vi "Read Data.vi"(8 "error in (no error)":errorcluster, 11 "Serial Config":T1={"串口选择"="", "通讯速率"=9600, "超时时间"=10000, "数据位长"=8, "奇偶校验"=enum."None", "停止位长"=10, "握手控制"=0, "字符结束"=TRUE, "结束字符"=10, "仪器地址"=1} {"结束字符" format="%.0x"; "握手控制" items=["None", "XON/XOFF", "RTS/CTS", "XON/XOFF & RTS/CTS", "DTR/DSR", "XON/XOFF & DTR/DSR"]; "停止位长" items=["1.0"=10, "1.5"=15, "2.0"=20]; "数据位长" min=5 max=8 step=1}) -> (0 "error out":errorcluster, 2 "Status":string, 3 "RV":dbl[](array[numeric]))   [LabVIEW 2010, in "CM51.lvlib"]
doc: "Use this template to build a VI to use as a subVI."
uses:
  CM51.lvlib
  Serial Config.ctl
  CM51Channel.ctl
  <vilib>/Instr/_visa.llb/VISA Configure Serial Port (Instr).vi
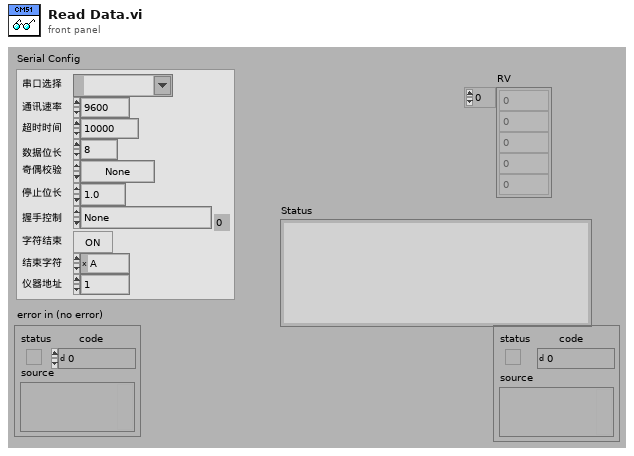
[diagram p1: front panel]
types:
  T1 = typedef "CM51.lvlib/Serial Config.ctl" = cluster{"串口选择":refnum<visa-resource-name>, "通讯速率":u32, "超时时间":u32, "数据位长":u16, "奇偶校验":enum16{"None", "Odd", "Even", "Mark", "Space"}, "停止位长":u16, "握手控制":u16, "字符结束":bool, "结束字符":u8, "仪器地址":u32}
  T2 = typedef "CM51.lvlib/CM51Channel.ctl" = enum16{"RV1", "RV2", "RV3"}
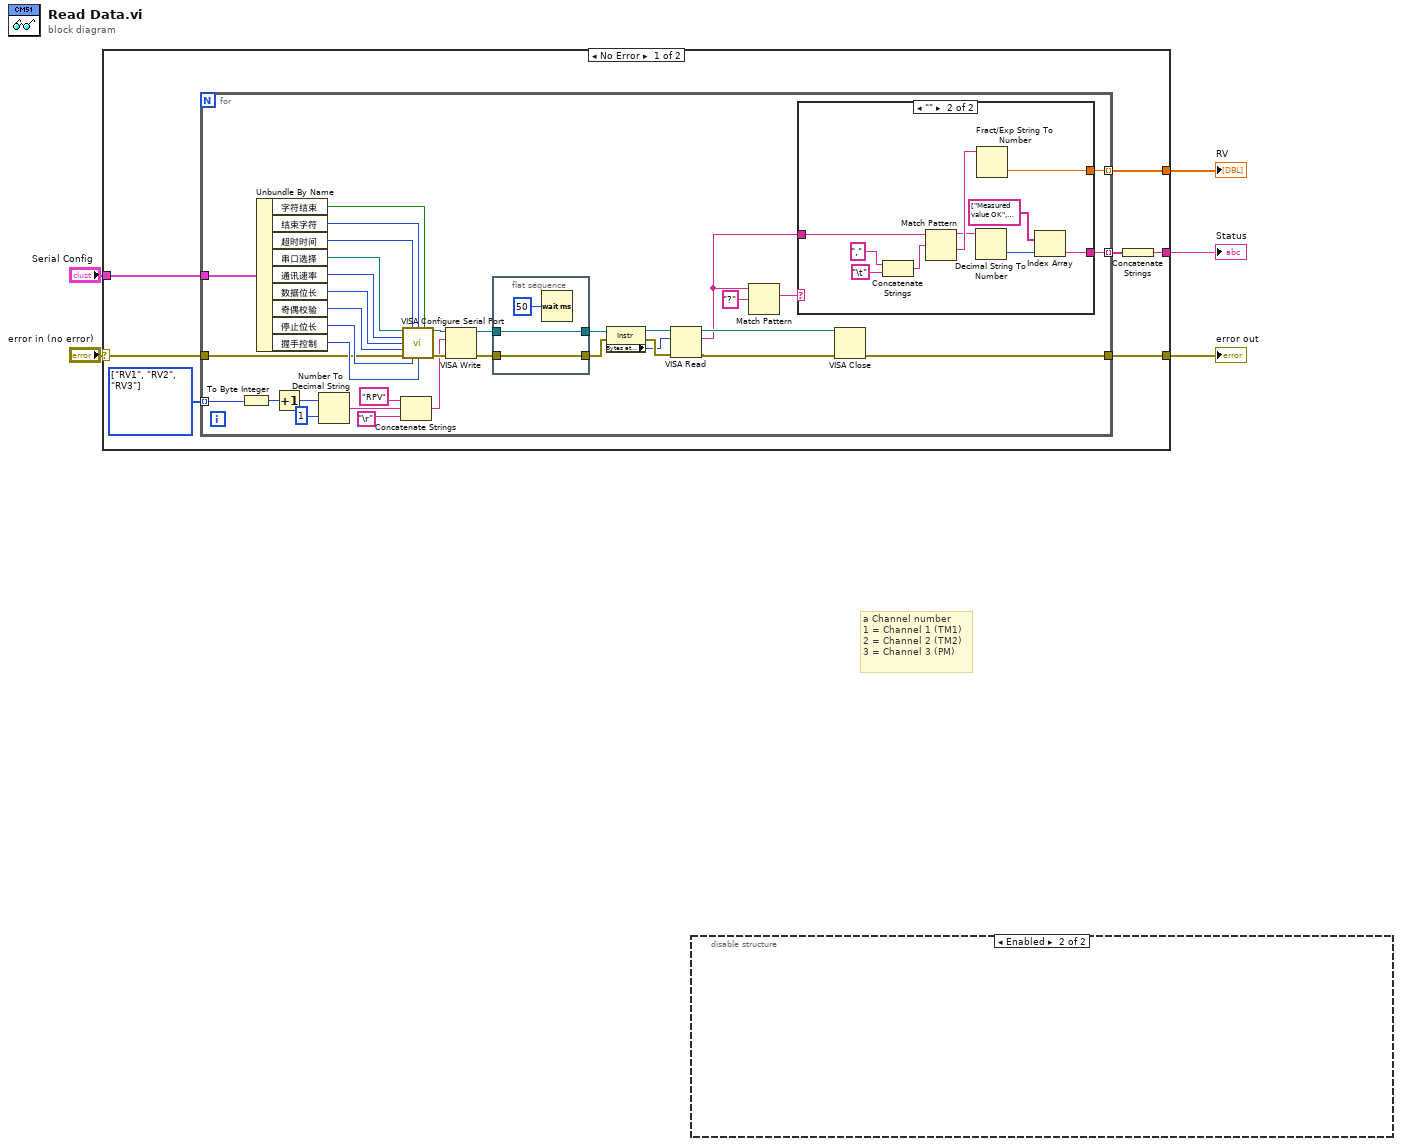
[diagram p0: block diagram]
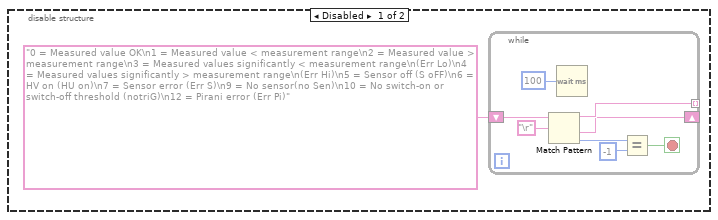
[diagram p2: hidden frame]
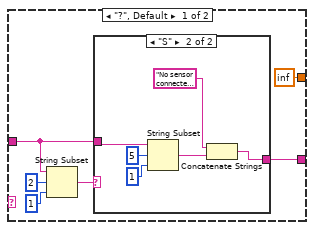
[diagram p3: hidden frame]
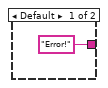
[diagram p4: hidden frame]
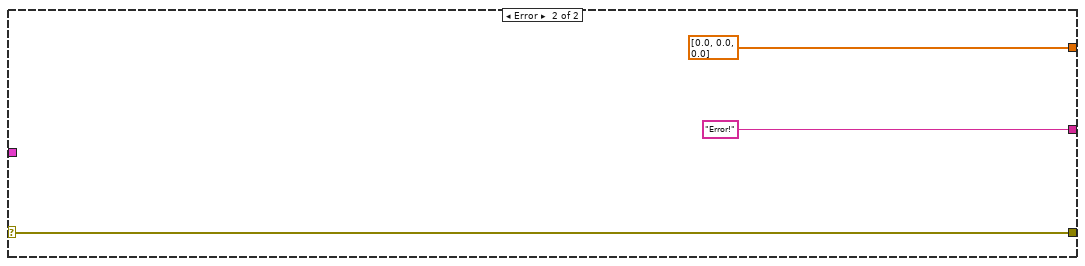
[diagram p5: hidden frame]
diagram:
  # "a Channel number\n1 = Channel 1 (TM1)\n2 = Channel 2 (TM2)\n3 = Channel 3 (PM)"
  n1 = case shown="No Error" "error in (no error)" {
    selector: "error in (no error)" -> [w11 w77]
    tunnel: [w10 w77] -> w4
    tunnel: "Serial Config" -> [w12 _]
    tunnel: [w6 "Error!"] -> w1
    tunnel: [w8 dbl[] [0.0, 0.0, 0.0]] -> w2
    frame No Error {
      w9 = T2[] [enum."RV1", enum."RV2", enum."RV3"] items=["RV1", "RV2", "RV3"]
      n2 = for {
        tunnel: w12 -> [w46]
        tunnel: w11 -> [w36]
        tunnel: [w35] -> w10
        tunnel: w9 -> [w28] mode=indexing
        tunnel: [w27] -> w7 mode=indexing
        tunnel: [w26] -> w8 mode=indexing
        n3 = To Byte Integer(number=w28) -> (8bit integer=w34:i8)
        n4 = Unbundle By Name(w46) -> ("字符结束"=w41:bool, "结束字符"=w42:u8, "超时时间"=w43:u32, "串口选择"=w45:refnum<visa-resource-name>, "通讯速率"=w44:u32, "数据位长"=w40:u16, "奇偶校验"=w39:enum16{"None", "Odd", "Even", "Mark", "Space"}, "停止位长"=w38:u16, "握手控制"=w37:u16)
        n5 = Increment(x=w34) -> (x+1=w33:i8)
        n6 = Number To Decimal String(number=w33, width (-)=i16 1 ("宽度(-)")) -> (decimal integer string=w30:string)
        n7 = Concatenate Strings("RPV" ("字符串"), w30, "\r") -> (w16:string)
        n8 = call-poly "VISA Configure Serial Port"("VISA resource name"=w45, "timeout (10sec)"=w43, "termination char\n(0xA = '\\n' = LF)"=w42, "Enable Termination\nChar (T)"=w41, "baud rate (9600)"=w44, "data bits (8)"=w40, "parity (0:none)"=w39, "error in (no error)"=w36, "stop bits (10: 1 bit)"=w38, "flow control (0:none)"=w37) -> ("VISA resource name out"=w47:refnum<visa-resource-name>, "error out"=w48:errorcluster)  [unwired: 4 in]
        n9 = VISA Write(VISA resource name=w47, write buffer=w16, error in (no error)=w48) -> (VISA resource name out=w20:refnum<visa-resource-name>, error out=w19:errorcluster)  [unwired: 1 out]
        n10 = flat-sequence {
          tunnel: w20 -> [w74]
          tunnel: w19 -> [w73]
          tunnel: [w74] -> w18
          tunnel: [w73] -> w17
          frame #0 {
            n11 = Wait (ms)(milliseconds to wait=u32 50) -> ()  [unwired: 1 out]
          }
        }
        n12 = property class="Instr"(reference=w18, error in=w17) -> (reference out=w25:refnum<visa-resource-name>, error out=w23:errorcluster, "Bytes at Port"=w22:u32)
        n13 = VISA Read(VISA resource name=w25, byte count=w22, error in (no error)=w23) -> (VISA resource name out=w24:refnum<visa-resource-name>, read buffer=w15:string, error out=w21:errorcluster)  [unwired: 1 out]
        n14 = Match Pattern(string=w15, regular expression="?") -> (match substring=w13:string)  [unwired: 1 in, 3 out]
        n15 = case shown="\"\"" w13 {
          tunnel: [w50 w70] -> w27
          tunnel: [inf w69] -> w26
          tunnel: w15 -> [w49 w62]
          frame "?", Default {
            n16 = String Subset(string=w49, offset (0)=2, length (rest)=1 ("length (rest)")) -> (substring=w52:string)
            n17 = case shown="\"S\"" w52 {
              tunnel: ["Error!" w56] -> w50
              tunnel: w49 -> [_ w59]
              frame Default {
              }
              frame "S" {
                n18 = String Subset(string=w59, offset (0)=5, length (rest)=1 ("length (rest)")) -> (substring=w57:string)
                n19 = Concatenate Strings("No sensor connected to channel ", w57) -> (w56:string)
              }
            }
          }
          frame "" {
            n20 = Concatenate Strings("," ("正则表达式"), "\t") -> (w65:string)
            n21 = Match Pattern(string=w62, regular expression=w65) -> (before substring=w66:string, after substring=w71:string)  [unwired: 1 in, 2 out]
            n22 = Decimal String To Number(string=w66) -> (number=w68:i32)  [unwired: 2 in, 1 out]
            n23 = Fract/Exp String To Number(string=w71) -> (number=w69:dbl)  [unwired: 3 in, 1 out]
            n24 = Index Array(array=string[] ["Measured value OK", "Measured value < measurement range", "Measured value > measurement range", "Measured values significantly < measurement range(Err Lo)", "Measured values significantly > measurement range(Err Hi)", "Sensor off (S oFF)", "HV on (HU on)", "Sensor error (Err S)", "No Define", "No sensor(no Sen)", "No switch-on or switch-off threshold (notriG)", "No Define", "Pirani error (Err Pi)", "\n"] ("通讯状态"), index=w68) -> (element=w70:string)
          }
        }
        n25 = VISA Close(VISA resource name=w24, error in (no error)=w21) -> (error out=w35:errorcluster)
      }
      n26 = Concatenate Strings(w7) -> (w6:string)
    }
    frame Error {
    }
  }
  "error out" <- w4
  "Status" <- w1
  "RV" <- w2
  n27 = disable-structure shown="Enabled" {
    frame Disabled {
      n28 = while {
        tunnel: [w86] -> _ mode=indexing
        shift-right: [w82] -> _
        shift-left: "0 = Measured value OK\n1 = Measured value < measurement range\n2 = Measured value > measurement range\n3 = Measured values significantly < measurement range\n(Err Lo)\n4 = Measured values significantly > measurement range\n(Err Hi)\n5 = Sensor off (S oFF)\n6 = HV on (HU on)\n7 = Sensor error (Err S)\n9 = No sensor(no Sen)\n10 = No switch-on or switch-off threshold (notriG)\n12 = Pirani error (Err Pi)" -> [w81]
        stop <- w83 stop-if-true
        n29 = Match Pattern(string=w81, regular expression="\r") -> (before substring=w86:string, after substring=w82:string, offset past match=w85:i32)  [unwired: 1 in, 1 out]
        n30 = Wait (ms)(milliseconds to wait=u32 100 ("等待时间（毫秒）")) -> ()  [unwired: 1 out]
        n31 = Equal?(x=w85, y=-1) -> (x = y?=w83:bool)
      }
    }
    frame Enabled {
    }
  }
